vi "Check_for_trigger.vi"(10 "Current trig":dbl, 11 "Plant":u16(ring) items=["Plant 1"=1, "Plant 2"=2]) -> (2 "Trigg'd?":bool, 3 "Bus data":dbl)   [LabVIEW 2016]
uses:
  <vilib>/xnet/xnet.llb/XNET Read (Signal Single-point).vi
panel:
  out "error out":errorcluster
  in  "error in (no error)":errorcluster
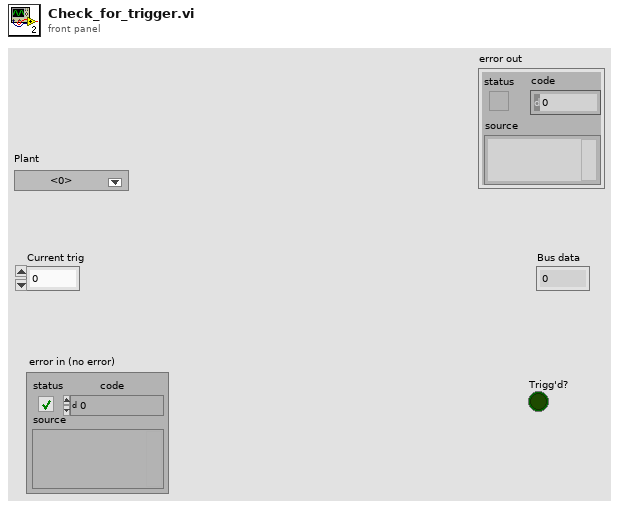
[diagram p1: front panel]
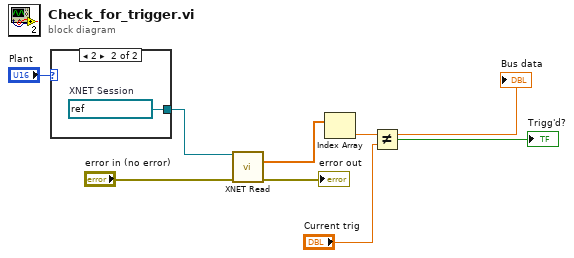
[diagram p0: block diagram]
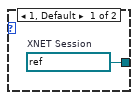
[diagram p2: hidden frame]
diagram:
  n1 = case shown="2" "Plant" {
    tunnel: [w9 w10] -> w2
    frame 1, Default {
      w9 = refnum<k21> "Plant1_trig"  # XNET Session
    }
    frame 2 {
      w10 = refnum<k21> "Plant2_trig"  # XNET Session
    }
  }
  n2 = call-poly <vilib>:"XNET Read.vi"("session in"=w2, "error in (no error)"="error in (no error)") -> ("data"=w6:dbl[], "error out"=→"error out":errorcluster)  [unwired: 11 in, 1 out]
  n3 = Index Array(array=w6) -> (element=w7:dbl)  [unwired: 1 in]
  "Bus data" <- w7
  n4 = Not Equal?(x=w7, y="Current trig") -> (x != y?=→"Trigg'd?":bool)
